vi "ExampleMeasurementServer.vi"() -> ()   [LabVIEW 2019]
uses:
  VIs/MeasurementServer_gRPCid.ctl
  Labview-lrms-proof-of-concept/Tesla-LRMS-PoC/JSONDefaults.ctl
  Labview-lrms-proof-of-concept/Tesla-LRMS-PoC/Global Operations.ctl
  VIs/labview-grpc-measurement-server.lvlib
panel:
  in  "Server Key File (.key)":path
  in  "Server Certificate File (.crt)":path
  in  "stop":bool
  in  "Server Address":string="0.0.0.0:50051"
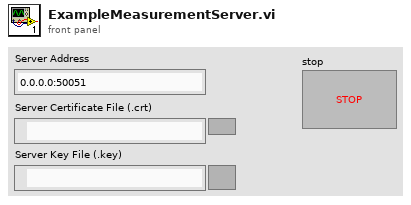
[diagram p1: front panel]
types:
  T1 = typedef "labview-grpc-measurement-server.lvlib/MeasurementServer_gRPCid.ctl" = u64
  T2 = cluster{"QueryServer_Invoke":refnum<user-event>, "QueryServer_Query":refnum<user-event>, "QueryServer_Register":refnum<user-event>, "QueryServer_FourProbeMeasurement":refnum<user-event>, "QueryServer_StreamFourProbeMeasurement":refnum<user-event>, "QueryServer_SendConfig":refnum<user-event>, "QueryServer_StreamError":refnum<user-event>, "gRPCid":T1}
  T3 = typedef "JSONDefaults.ctl" = string[]
  T4 = typedef "Global Operations.ctl" = enum16{"Get", "Set"}
  T5 = typedef "labview-grpc-measurement-server.lvlib/MeasurementServer_ConfigRequest.ctl" = cluster{"SMUResourceName":string, "SMUChannels":string, "SMUSourceMode":i32, "SMUOutputFunction":i32, "SMUSourceTransientResponse":i32, "SMUCurrent":sgl, "SMUCurrentLevelRange":sgl, "SMUMeasurementSense":i32, "SMUMeasurementApertureTime":sgl, "SMUSourceAdvancedSourceDelay":sgl, "SMUVoltage":sgl, "SMUSourceAdvancedSequenceLoopCount":i32, "SMUMeasurementAdvancedDCNoiseRejection":i32, "SMUSequenceName":string, "ScanList":string, "DMMResourceName":string, "DMMFunction":i32, "DMMResolution":sgl, "DMMRange":sgl, "DMMSampleCount":i32, "DMMApertureTimeUnit":i32, "DMMApertureTime":sgl, "DMMNumberOfAverages":i32, "DMMAutoZero":i32, "DMMADCCalibration":i32, "DMMSettleTime":sgl, "DMMControlAction":i32, "DMMVoltageFaultUpperLimit":sgl, "ApplicationNumberOfWeldChannels":i32}
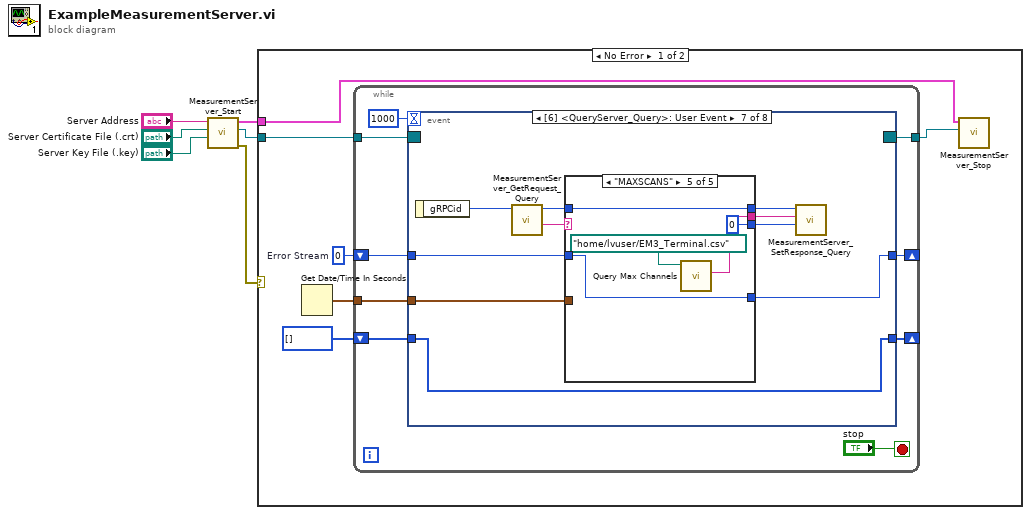
[diagram p0: block diagram]
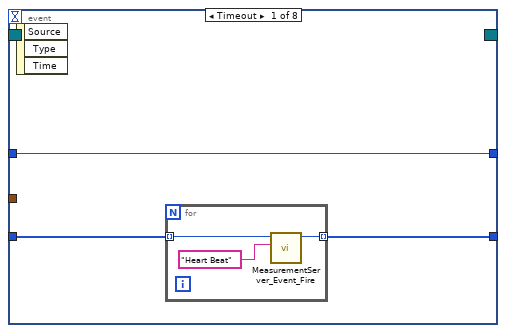
[diagram p2: hidden frame]
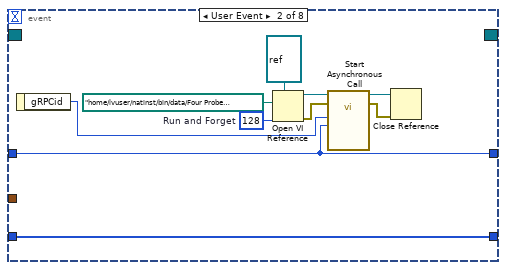
[diagram p3: hidden frame]
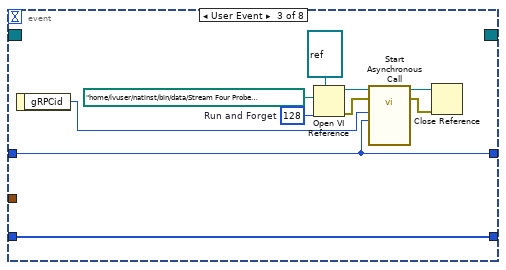
[diagram p4: hidden frame]
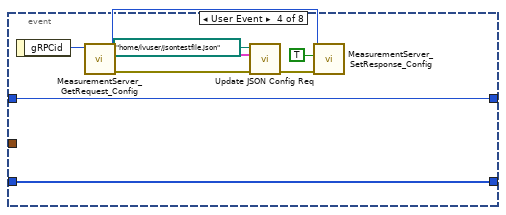
[diagram p5: hidden frame]
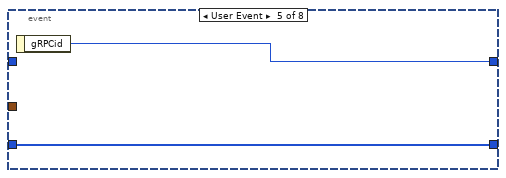
[diagram p6: hidden frame]
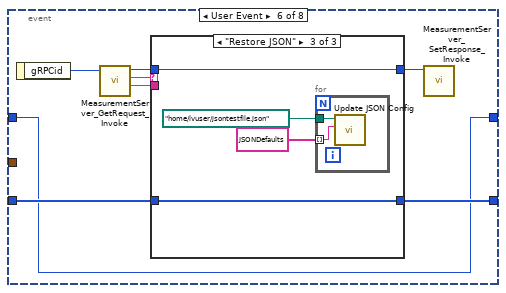
[diagram p7: hidden frame]
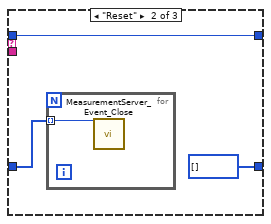
[diagram p9: hidden frame]
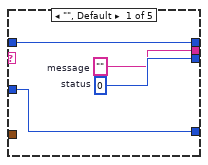
[diagram p10: hidden frame]
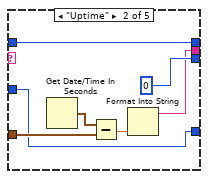
[diagram p11: hidden frame]
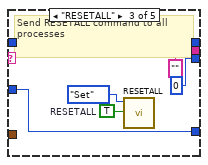
[diagram p12: hidden frame]
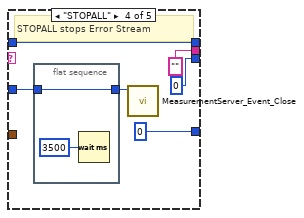
[diagram p13: hidden frame]
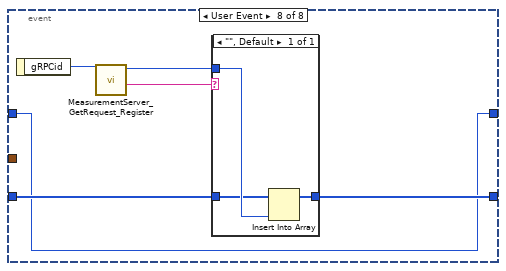
[diagram p14: hidden frame]
diagram:
  n1 = call "MeasurementServer_Start.vi"("Server Key File (.key)"="Server Key File (.key)", "Server Certificate File (.crt)"="Server Certificate File (.crt)", "Server Address"="Server Address") -> ("error out"=w2:errorcluster, "Event Registration Refnum"=w1:refnum<event-registration>, "Server Information"=w5:T2)  [unwired: 5 in]
  n2 = case shown="No Error" w2 {
    tunnel: w5 -> [w10 _]
    tunnel: w1 -> [w9 _]
    frame No Error {
      w7 = T1 0  # Error Stream
      n3 = Get Date/Time In Seconds() -> (seconds since 1Jan1904=w12:timestamp)
      n4 = while {
        tunnel: [w20] -> w8
        tunnel: w12 -> [w19]
        shift-right: [w17] -> _
        shift-left: u64[] [] -> [w16]
        tunnel: w9 -> [w15]
        shift-right: [w14] -> _
        shift-left: w7 -> [w13]
        stop <- "stop" stop-if-true
        n5 = event shown="[6] <QueryServer_Query>: User Event" {
          selector: w15 -> [_ _ _ _ _ _ _ _]
          dyn-events: [_ _ _ _ _ _ _ _] -> w20
          timeout: 1000 -> [_ _ _ _ _ _ _ _]
          tunnel: w19 -> [_ _ _ _ _ _ w84 _]
          tunnel: [w24 w37 w38 w53 w57 w60 w83 w122] -> w17
          tunnel: w16 -> [w23 w37 w38 w53 w57 w61 w83 w121]
          tunnel: [w22 w30 w39 w52 w58 w59 w80 w119] -> w14
          tunnel: w13 -> [w22 w30 w39 w52 _ w59 w81 w119]
          event Timeout {
            n6 = event-data() -> ()  [unwired: 1 in, 3 out]
            n7 = for {
              tunnel: w23 -> [w27] mode=indexing
              tunnel: [w25] -> w24 mode=indexing
              n8 = call "MeasurementServer_Event_Fire.vi"("eventdata"="Heart Beat", "gRPCid"=w27) -> ("gRPCid out"=w25:T1)  [unwired: 8 in, 1 out]
            }
          }
          event User Event {
            w35 = 128  # Run and Forget
            n9 = event-data() -> ("gRPCid"=w31:T1)  [unwired: 1 in]
            n10 = Open VI Reference(type specifier VI Refnum (for type only)=refnum<vi> refnum, vi path=path "/home/lvuser/natinst/bin/data/Four Probe Asynchronous.vi", options=w35) -> (vi reference=w33:refnum<vi>, error out=w32:errorcluster)  [unwired: 3 in]
            n11 = call-by-ref "Start Asynchronous Call"(reference=w33, error in=w32, "Error Stream gRPCid"=w30, "gRPCid"=w31) -> (reference out=w28:refnum<vi>, error out=w29:errorcluster)  [unwired: 10 in]
            n12 = Close Reference(reference=w28, error in (no error)=w29) -> ()  [unwired: 1 out]
          }
          event User Event {
            w46 = 128  # Run and Forget
            n13 = event-data() -> ("gRPCid"=w40:T1)  [unwired: 1 in]
            n14 = Open VI Reference(type specifier VI Refnum (for type only)=refnum<vi> refnum, vi path=path "/home/lvuser/natinst/bin/data/Stream Four Probe Asynchronous.vi", options=w46) -> (vi reference=w44:refnum<vi>, error out=w43:errorcluster)  [unwired: 3 in]
            n15 = call-by-ref "Start Asynchronous Call"(reference=w44, error in=w43, "Error Stream gRPCid"=w39, "gRPCid"=w40) -> (reference out=w41:refnum<vi>, error out=w42:errorcluster)  [unwired: 10 in]
            n16 = Close Reference(reference=w41, error in (no error)=w42) -> ()  [unwired: 1 out]
          }
          event User Event {
            n17 = event-data() -> ("gRPCid"=w56:T1)  [unwired: 1 in]
            n18 = call "MeasurementServer_GetRequest_Config.vi"("gRPCid"=w56) -> ("error out"=w50:errorcluster, "ConfigRequest"=w48:T5, "gRPCid out"=w55:T1)  [unwired: 6 in]
            n19 = call "Update JSON Config Req.vi"("error in (no error)"=w50, "ConfigRequest"=w48, "JSON Configuration File (.json)"=path "/home/lvuser/jsontestfile.json") -> ("error out"=w49:errorcluster)  [unwired: 8 in]
            n20 = call "MeasurementServer_SetResponse_Config.vi"("gRPCid"=w55, "acknowledge"=TRUE, "error in (no error)"=w49) -> ()  [unwired: 7 in, 1 out]
          }
          event User Event {
            n21 = event-data() -> ("gRPCid"=w58:T1)  [unwired: 1 in]
          }
          event User Event {
            n22 = event-data() -> ("gRPCid"=w66:T1)  [unwired: 1 in]
            n23 = call "MeasurementServer_GetRequest_Invoke.vi"("gRPCid"=w66) -> ("parameter"=w62:string, "command"=w65:string, "gRPCid out"=w64:T1)  [unwired: 5 in, 1 out]
            n24 = case shown="\"Restore JSON\"" w65 {
              tunnel: w64 -> [w68 w69 w74]
              tunnel: [w68 w69 w74] -> w63
              tunnel: w62 -> [_ _ _]
              tunnel: w61 -> [w67 w71 w73]
              tunnel: [w67 u64[] [] w73] -> w60
              frame "", Default {
              }
              frame "Reset" {
                n25 = for {
                  tunnel: w71 -> [w72] mode=indexing
                  n26 = call "MeasurementServer_Event_Close.vi"("gRPCid"=w72) -> ()  [unwired: 9 in, 1 out]
                }
              }
              frame "Restore JSON" {
                n27 = for {
                  tunnel: path "/home/lvuser/jsontestfile.json" ("JSON Configuration File (.json)") -> [w78]
                  tunnel: T3 ["SETCONF=SMUResourceName[[CONFPARAM]]=SMU", "SETCONF=SMUChannels[[CONFPARAM]]=0", "SETCONF=SMUSourceMode[[CONFPARAM]]=1021", "SETCONF=SMUOutputFunction[[CONFPARAM]]=1007", "SETCONF=SMUSourceTransientResponse[[CONFPARAM]]=1039", "SETCONF=SMUCurrent[[CONFPARAM]]=1.0", "SETCONF=SMUCurrentLevelRange[[CONFPARAM]]=1.0", "SETCONF=SMUMeasurementSense[[CONFPARAM]]=1008", "SETCONF=SMUMeasurementApertureTime[[CONFPARAM]]=0.010", "SETCONF=SMUSourceAdvancedSourceDelay[[CONFPARAM]]=0.000100", "SETCONF=SMUVoltage[[CONFPARAM]]=6", "SETCONF=SMUSourceAdvancedSequenceLoopCount[[CONFPARAM]]=571", "SETCONF=SMUMeasurementAdvancedDCNoiseRejection[[CONFPARAM]]=1044", "SETCONF=SMUSequenceName[[CONFPARAM]]=MySequence", "SETCONF=SMUStep1_Source_DCCurrent_CurrentLevel[[CONFPARAM]]=1150009", "SETCONF=SMUStep2_Measurement_ApertureTime[[CONFPARAM]]=1150058", "SETCONF=SMUStep3_Source_Advanced_SourceDelay[[CONFPARAM]]=1150051", "SETCONF=SMUSequenceNumberOfSteps[[CONFPARAM]]=3", "SETCONF=ScanList[[CONFPARAM]]=SCANALL", "SETCONF=Switch1ResourceName[[CONFPARAM]]=2526_1", "SETCONF=Switch1Topology[[CONFPARAM]]=2526/2-Wire 79x1 Mux", "SETCONF=Switch1ScanList[[CONFPARAM]]=ch70:75->com", "SETCONF=Switch2ResourceName[[CONFPARAM]]=SwitchBlock1Dev1", "SETCONF=Switch2Topology[[CONFPARAM]]=Configured Topology", "SETCONF=Switch2ScanList[[CONFPARAM]]=[c2->card1r2->c26], [c3->card1r3->c27]; [c6->card1r2->c26], [c7->card1r3->c27]; [c10->card1r2->c26], [c11->card1r3->c27]; [c14->card1r2->c26], [c15->card1r3->c27]; [c18->card1r2->c26], [c19->card1r3->c27]; [c22->card1r2->c26], [c23->card1r3->c27];", "SETCONF=DMMResourceName[[CONFPARAM]]=DMM", "SETCONF=DMMFunction[[CONFPARAM]]=0", "SETCONF=DMMResolution[[CONFPARAM]]=0.1", "SETCONF=DMMRange[[CONFPARAM]]=0.1", "SETCONF=DMMSampleCount[[CONFPARAM]]=0", "SETCONF=DMMApertureTimeUnit[[CONFPARAM]]=0", "SETCONF=DMMApertureTime[[CONFPARAM]]=0.010", "SETCONF=DMMNumberOfAverages[[CONFPARAM]]=1", "SETCONF=DMMAutoZero[[CONFPARAM]]=0", "SETCONF=DMMADCCalibration[[CONFPARAM]]=0", "SETCONF=DMMSettleTime[[CONFPARAM]]=0.0001", "SETCONF=DMMControlAction[[CONFPARAM]]=0", "SETCONF=DMMVoltageFaultUpperLimit[[CONFPARAM]]=0.000050", "SETCONF=ApplicationNumberOfWeldChannels[[CONFPARAM]]=6"] ("JSON Defaults") -> [w77] mode=indexing
                  n28 = call "Update JSON Config.vi"("Parameter and Value"=w77, "JSON Configuration File (.json)"=w78) -> ()  [unwired: 9 in, 1 out]
                }
              }
            }
            n29 = call "MeasurementServer_SetResponse_Invoke.vi"("gRPCid"=w63) -> ()  [unwired: 9 in, 1 out]
          }
          event User Event {
            n30 = event-data() -> ("gRPCid"=w88:T1)  [unwired: 1 in]
            n31 = call "MeasurementServer_GetRequest_Query.vi"("gRPCid"=w88) -> ("gRPCid out"=w87:T1, "query"=w82:string)  [unwired: 7 in, 1 out]
            n32 = case shown="\"MAXSCANS\"" w82 {
              tunnel: w87 -> [w92 w96 w105 w111 w118]
              tunnel: [w92 w96 w105 w111 w118] -> w86
              tunnel: [w91 0 ("status") 0 ("status") 0 ("status") 0 ("status")] -> w85
              tunnel: w84 -> [_ w98 _ _ _]
              tunnel: w81 -> [w90 w94 w101 w109 w117]
              tunnel: [w90 w94 w101 T1 0 ("Error Stream") w117] -> w80
              tunnel: [w89 w93 "" ("message") "" ("message") w114] -> w79
              frame "", Default {
                w91 = 0  # status
                w89 = ""  # message
              }
              frame "Uptime" {
                n33 = Get Date/Time In Seconds() -> (seconds since 1Jan1904=w99:timestamp)
                n34 = Subtract(x=w99, y=w98) -> (x-y=w97:dbl)
                n35 = Format Into String(w97) -> (resulting string=w93:string)  [unwired: 3 in, 1 out]
              }
              frame "RESETALL" {
                w102 = TRUE  # RESETALL
                # "Send RESETALL command to all processes"
                n36 = call "RESETALL.vi"("RESETALL"=w102, "Operation"=Global_Operations."Set" ("Enum")) -> ()  [unwired: 8 in, 2 out]
              }
              frame "STOPALL" {
                # "STOPALL stops Error Stream"
                n37 = flat-sequence {
                  tunnel: w109 -> [w113]
                  tunnel: [w113] -> w107
                  frame #0 {
                    n38 = Wait (ms)(milliseconds to wait=u32 3500) -> ()  [unwired: 1 out]
                  }
                }
                n39 = call "MeasurementServer_Event_Close.vi"("gRPCid"=w107) -> ()  [unwired: 9 in, 1 out]
              }
              frame "MAXSCANS" {
                n40 = call "Query Max Channels.vi"("file path (dialog if empty)"=path "/home/lvuser/EM3_Terminal.csv") -> ("Num channels"=w114:string)  [unwired: 9 in, 1 out]
              }
            }
            n41 = call "MeasurementServer_SetResponse_Query.vi"("gRPCid"=w86, "message"=w79, "status"=w85) -> ()  [unwired: 7 in, 1 out]
          }
          event User Event {
            n42 = event-data() -> ("gRPCid"=w124:T1)  [unwired: 1 in]
            n43 = call "MeasurementServer_GetRequest_Register.vi"("gRPCid"=w124) -> ("gRPCid out"=w123:T1, "eventname"=w120:string)  [unwired: 7 in, 1 out]
            n44 = case shown="\"\", Default" w120 {
              tunnel: w123 -> [w127]
              tunnel: [w126] -> w122
              tunnel: w121 -> [w125]
              frame "", Default {
                n45 = Insert Into Array(array=w125, new element=w127) -> (w126:T1[])  [unwired: 1 in]
              }
            }
          }
        }
      }
      n46 = call "MeasurementServer_Stop.vi"("Server Information"=w10, "Event Registration Refnum"=w8) -> ()  [unwired: 8 in, 1 out]
    }
    frame Error {
    }
  }
